vi "Obtain Thread.vi"(8 "error in (no error)":errorcluster, 11 "Plugin in":refnum<class "Plugin.lvclass">) -> (0 "error out":errorcluster, 2 "Plugin Thread Interface":refnum<class "Plugin Interface.lvclass">, 3 "Plugin out":refnum<class "Plugin.lvclass">)   [LabVIEW 2017, in "DSF Core.lvlib" / "Plugin.lvclass"]
uses:
  Plugin.lvclass
  Interfaces/Transceiver Interface/Plugin Interface.lvclass
  Plugin.lvclass/Plugin.ctl
  Thread Pool/Pool.lvclass/Pool.ctl
  Debug/FIFO Flags/FIFO Flags.lvclass/FIFO Flags.ctl
  Thread Pool/Read FIFO.vi
  Thread Pool/Get FIFO.vi
  Thread Pool/Get Debug Flags.vi
  Debug/FIFO Flags/Get Infinite Timeouts.vi
  Thread Pool/ID Pool.lvclass
  C:/Git/DSF/Data Sharing Framework/Source/Core/Engine/Classes/Thread Pool/Pool.lvclass
  Thread Pool/Errors.vi
  Thread Pool/Obtain ID Timeout.vi
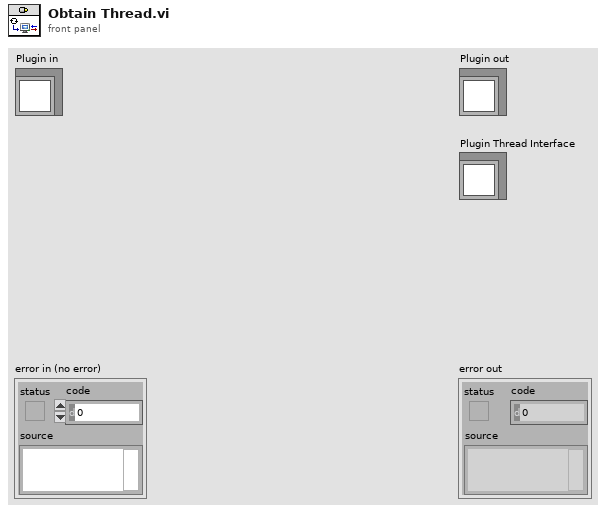
[diagram p1: front panel]
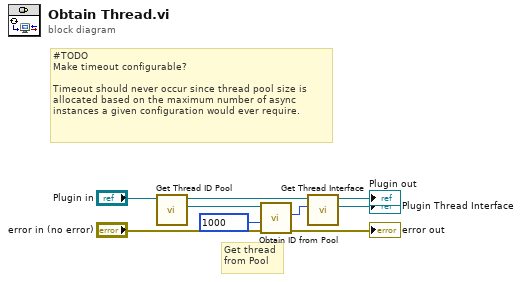
[diagram p0: block diagram]
diagram:
  # "#TODO\nMake timeout configurable?\n\nTimeout should never occur since thread pool size is allocated based on the maximum number of async instances a given configuration would ever require."
  # "Get thread from Pool"
  n1 = call "Get Thread ID Pool.vi"("Plugin in"="Plugin in") -> ("Thread ID Pool"=w7:refnum<class "ID Pool.lvclass">, "Plugin out"=w5:refnum<class "Plugin.lvclass">)  [unwired: 9 in]
  n2 = call "Obtain ID from Pool.vi"("error in (no error)"="error in (no error)", "timeout in ms (0)"=1000, "ID Pool in"=w7) -> ("error out"=→"error out":errorcluster, "id"=w4:i32)  [unwired: 5 in, 2 out]
  n3 = call "Get Thread Interface.vi"("index"=w4, "Plugin in"=w5) -> ("Plugin Interface"=→"Plugin Thread Interface":refnum<class "Plugin Interface.lvclass">, "Plugin out"=→"Plugin out":refnum<class "Plugin.lvclass">)  [unwired: 8 in]
